vi "Quick Sort 3D Coordinates.vi"(4 "3D Coordinates":cluster{"x1":dbl, "x2":dbl, "x3":dbl}[](array[cluster])) -> (1 "Sorted 3D Coordinates":cluster{"x1":dbl, "x2":dbl, "x3":dbl}[](array[cluster]))   [LabVIEW 2013]
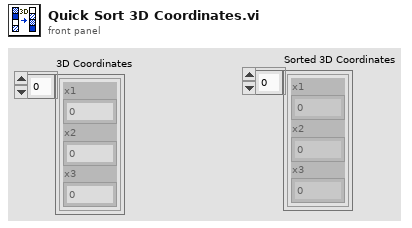
[diagram p1: front panel]
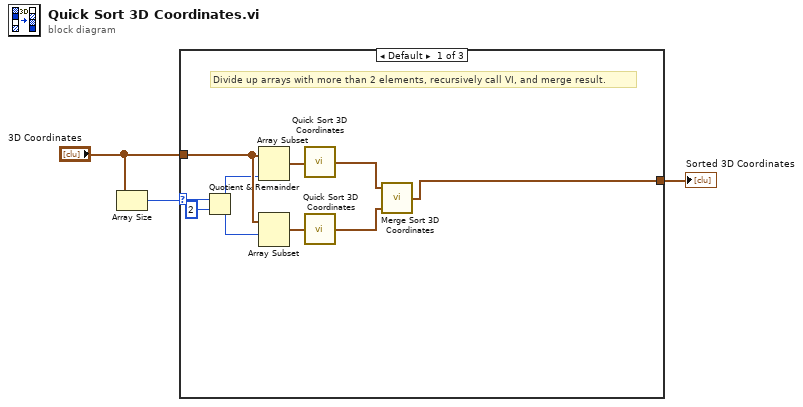
[diagram p0: block diagram]
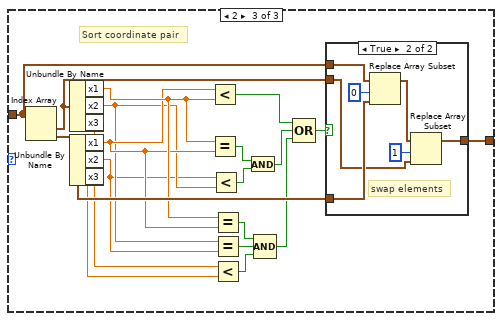
[diagram p3: hidden frame]
diagram:
  n1 = Array Size(array="3D Coordinates") -> (size(s)=w3:i32)
  n2 = case shown="Default" w3 {
    selector: w3 -> [w12 _ _]
    tunnel: "3D Coordinates" -> [w10 w13 w27]
    tunnel: [w4 w13 w25] -> w1
    frame Default {
      # "Divide up arrays with more than 2 elements, recursively call VI, and merge result."
      n3 = Quotient & Remainder(x=w12, y=2) -> (floor(x/y)=w9:i32)  [unwired: 1 out]
      n4 = Array Subset(array=w10, length=w9) -> (w8:cluster{"x1":dbl, "x2":dbl, "x3":dbl}[])  [unwired: 1 in]
      n5 = Array Subset(array=w10, index=w9) -> (w7:cluster{"x1":dbl, "x2":dbl, "x3":dbl}[])  [unwired: 1 in]
      n6 = call "Quick Sort 3D Coordinates.vi"("3D Coordinates"=w8) -> ("Sorted 3D Coordinates"=w6:cluster{"x1":dbl, "x2":dbl, "x3":dbl}[])  [unwired: 4 in]
      n7 = call "Quick Sort 3D Coordinates.vi"("3D Coordinates"=w7) -> ("Sorted 3D Coordinates"=w5:cluster{"x1":dbl, "x2":dbl, "x3":dbl}[])  [unwired: 4 in]
      n8 = call "Merge Sort 3D Coordinates.vi"("3D Coordinates B"=w5, "3D Coordinates A"=w6) -> ("Sorted 3D Coordinates"=w4:cluster{"x1":dbl, "x2":dbl, "x3":dbl}[])  [unwired: 3 in]
    }
    frame 0, 1 {
      # "Pass through single elements."
    }
    frame 2 {
      # "Sort coordinate pair"
      n9 = Index Array(array=w27) -> (element #1=w26:cluster{"x1":dbl, "x2":dbl, "x3":dbl}, element #2=w28:cluster{"x1":dbl, "x2":dbl, "x3":dbl})  [unwired: 2 in]
      n10 = Unbundle By Name(w26) -> ("x1"=w19:dbl, "x2"=w17:dbl, "x3"=w15:dbl)
      n11 = Unbundle By Name(w28) -> ("x1"=w18:dbl, "x2"=w16:dbl, "x3"=w14:dbl)
      n12 = Less?(x=w18, y=w19) -> (x < y?=w32:bool)
      n13 = Equal?(x=w19, y=w18) -> (x = y?=w31:bool)
      n14 = Less?(x=w16, y=w17) -> (x < y?=w30:bool)
      n15 = Equal?(x=w19, y=w18) -> (x = y?=w23:bool)
      n16 = Equal?(x=w17, y=w16) -> (x = y?=w20:bool)
      n17 = Less?(x=w14, y=w15) -> (x < y?=w21:bool)
      n18 = And(x=w31, y=w30) -> (x .and. y?=w29:bool)
      n19 = Compound Arithmetic op=AND(w23, w20, w21) -> (w22:bool)
      n20 = Compound Arithmetic op=OR(w32, w29, w22) -> (w24:bool)
      n21 = case shown="True" w24 {
        tunnel: w28 -> [_ w39]
        tunnel: w27 -> [w33 w38]
        tunnel: w26 -> [_ w36]
        tunnel: [w33 w34] -> w25
        frame False {
        }
        frame True {
          # "swap elements"
          n22 = Replace Array Subset(array=w38, new element=w39, index=0) -> (w35:cluster{"x1":dbl, "x2":dbl, "x3":dbl}[])
          n23 = Replace Array Subset(array=w35, new element=w36, index=1) -> (w34:cluster{"x1":dbl, "x2":dbl, "x3":dbl}[])
        }
      }
    }
  }
  "Sorted 3D Coordinates" <- w1
